vi "Snap Frame.vi"(8 "error in (no error)":errorcluster, 9 "Imaq Image pointer":T1, 10 "Camera State In":T2 {"Sub Region"."V Size"."Value" min=0 max=0 step=4; "Sub Region"."H Size"."Value" min=0 max=0 step=4; "Sub Region"."V Offset"."Value" min=0 max=0 step=4; "Sub Region"."H Offset"."Value" min=0 max=0 step=4}, 11 "Image Data Notifier":refnum<notifier>) -> (0 "error in (no error) 2":errorcluster, 1 "Data Out":u16[][](array[numeric]), 2 "Camera State Out":T2 {"Sub Region"."V Size"."Value" min=0 max=0 step=4; "Sub Region"."H Size"."Value" min=0 max=0 step=4; "Sub Region"."V Offset"."Value" min=0 max=0 step=4; "Sub Region"."H Offset"."Value" min=0 max=0 step=4}, 3 "Done?":bool)   [LabVIEW 2015, in "Camera.lvlib"]
uses:
  Camera.lvlib
  Camera State.ctl
  Camera Loop State.ctl
  <vilib>/Utility/miscctls.llb/LVMinMaxIncTypeDef.ctl
  Acquisition Settings.ctl
  Live View State.ctl
  <vilib>/vision/Image Controls.llb/IMAQ Image.ctl
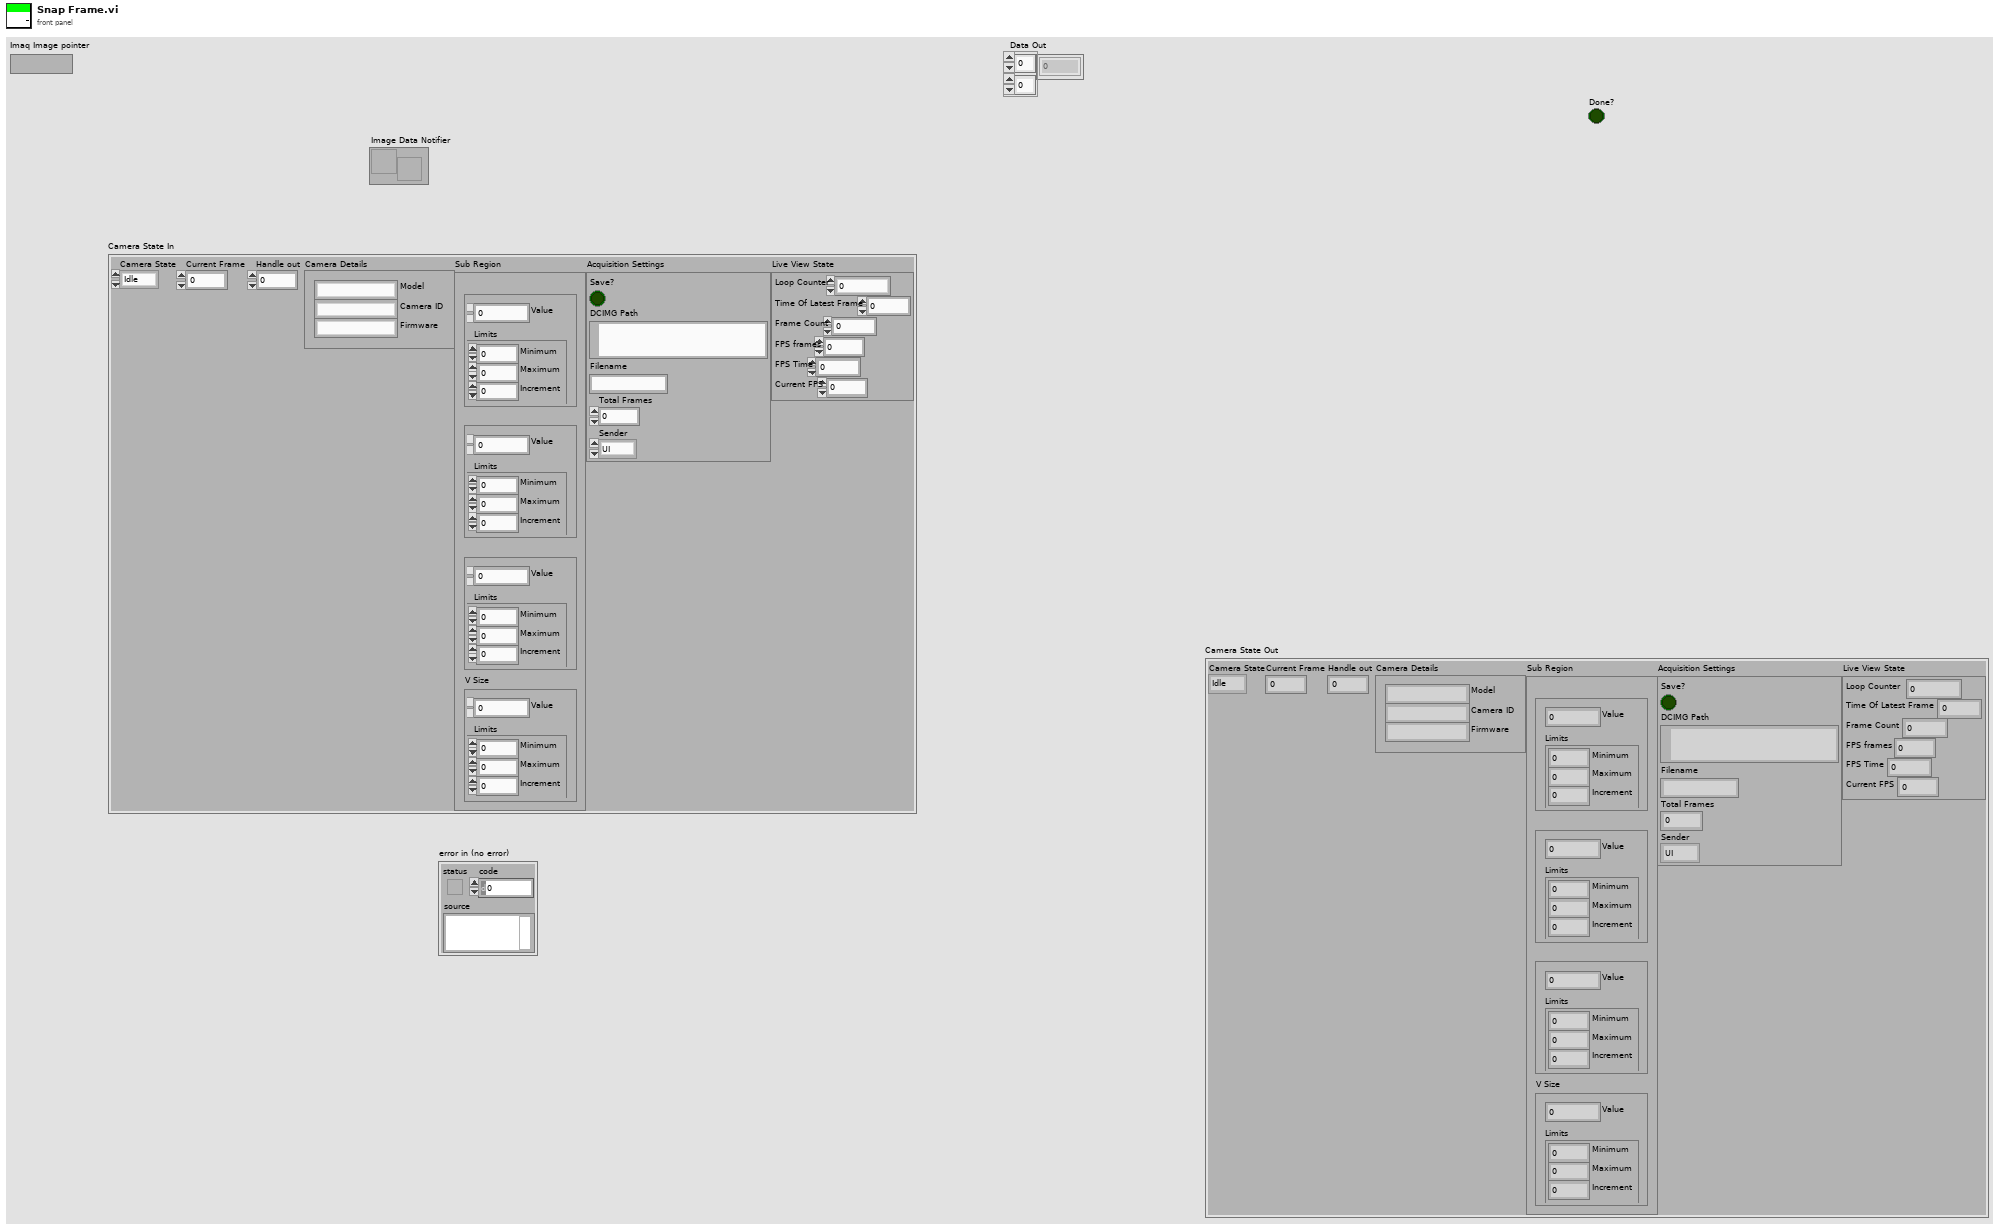
[diagram p1: front panel]
types:
  T1 = typedef "IMAQ Image.ctl" = refnum<image>
  T2 = typedef "Camera.lvlib/Camera State.ctl" = cluster{"Camera State":T3, "Current Frame":i32, "Handle out":u32, "Camera Details":cluster{"Model":string, "Camera ID":string, "Firmware":string}, "Sub Region":cluster{"H Offset":cluster{"Value":i32, "Limits":T4}, "V Offset":cluster{"Value":i32, "Limits":T4}, "H Size":cluster{"Value":i32, "Limits":T4}, "V Size":cluster{"Value":i32, "Limits":T4}}, "Acquisition Settings":T5, "Live View State":T6}
  T3 = typedef "Camera.lvlib/Camera Loop State.ctl" = enum16{"Idle", "Live View", "Ready", "Acquiring"}
  T4 = typedef "LVMinMaxIncTypeDef.ctl" = cluster{"Minimum":dbl, "Maximum":dbl, "Increment":dbl}
  T5 = typedef "Camera.lvlib/Acquisition Settings.ctl" = cluster{"Save?":bool, "DCIMG Path":path, "Filename":string, "Total Frames":i32, "Sender":enum16{"UI", "Automation"}}
  T6 = typedef "Camera.lvlib/Live View State.ctl" = cluster{"Loop Counter":i32, "Time Of Latest Frame":u32, "Frame Count":u32, "FPS frames":dbl, "FPS Time":u32, "Current FPS":dbl}
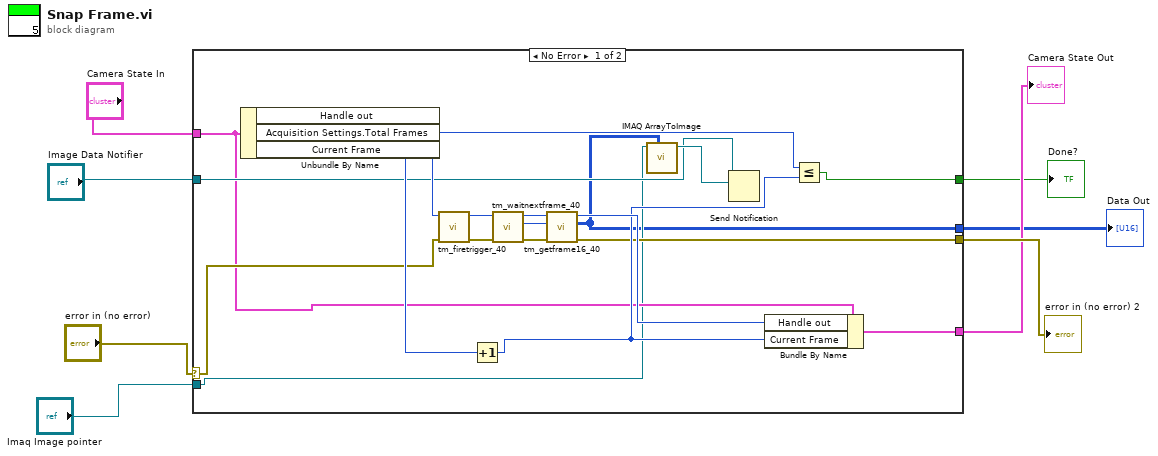
[diagram p0: block diagram]
diagram:
  n1 = case shown="No Error" "error in (no error)" {
    selector: "error in (no error)" -> [w15 w28]
    tunnel: "Camera State In" -> [w14 _]
    tunnel: "Image Data Notifier" -> [w16 _]
    tunnel: [w13 w28] -> w5
    tunnel: "Imaq Image pointer" -> [w12 _]
    tunnel: [w11 _] -> w3
    tunnel: [w10 _] -> w2
    tunnel: [w9 _] -> w1
    frame No Error {
      n2 = Unbundle By Name(w14) -> ("Handle out"=w22:u32, "Acquisition Settings.Total Frames"=w19:i32, "Current Frame"=w21:i32)
      n3 = call <userlib>:"tm_firetrigger_40.vi"("error in (no error)"=w15, "Handle in"=w22) -> ("error out"=w24:errorcluster, "Handle out"=w25:u32)  [unwired: 8 in]
      n4 = Increment(x=w21) -> (x+1=w18:i32)
      n5 = call <userlib>:"tm_waitnextframe_40.vi"("error in (no error)"=w24, "Handle in"=w25) -> ("error out"=w27:errorcluster, "Frame Index"=w23:i32, "Handle out"=w26:u32)  [unwired: 6 in, 1 out]
      n6 = call <userlib>:"tm_getframe16_40.vi"("error in (no error)"=w27, "Frame Index"=w23, "Handle in"=w26) -> ("error out"=w13:errorcluster, "Data"=w9:u16[][], "Handle out"=w20:u32)  [unwired: 5 in, 1 out]
      n7 = call "IMAQ ArrayToImage"("Image Pixels (U16)"=w9, "Image"=w12) -> ("Image Out"=w17:T1)  [unwired: 8 in, 1 out]
      n8 = Send Notification(notification=w17, notifier=w16) -> ()  [unwired: 1 in, 2 out]
      n9 = Bundle By Name(cluster=w14, "Handle out"=w20, "Current Frame"=w18) -> (w11:T2)
      n10 = Less Or Equal?(x=w19, y=w18) -> (x <= y?=w10:bool)
    }
    frame Error {
    }
  }
  "error in (no error) 2" <- w5
  "Camera State Out" <- w3
  "Done?" <- w2
  "Data Out" <- w1
